vi "Read Configuration Parameters.vi"(8 "error in (no error)":errorcluster, 10 "refnum":T1, 11 "UserPwd DB Configuration in":refnum<class "UserPwd DB Configuration.lvclass">) -> (0 "error out":errorcluster, 2 "refnum out":T1, 3 "UserPwd DB Configuration out":refnum<class "UserPwd DB Configuration.lvclass">)   [LabVIEW 2016, in "UserPwd DB.lvlib" / "UserPwd DB Configuration.lvclass"]
uses:
  <userlib>/Common Components/UserPwd DB/UserPwd DB Config/UserPwd DB Configuration.lvclass
  <vilib>/Utility/config.llb/Config Data RefNum.ctl
  <userlib>/Common Components/UserPwd DB/UserPwd DB/UserPwd DB.lvclass
  <userlib>/Common Components/UserPwd DB/UserPwd DB Config/UserPwd DB Configuration.lvclass/UserPwd DB Configuration.ctl
  <userlib>/Configuration Dialog Actor/Configuration.lvclass
  <vilib>/Utility/config.llb/NI_LVConfig.lvlib
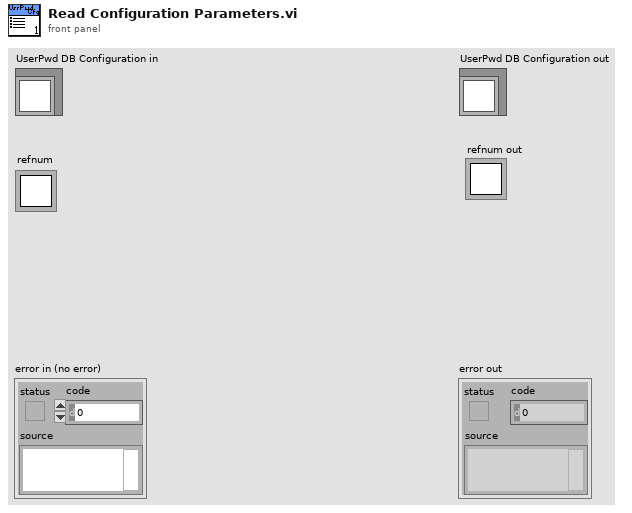
[diagram p1: front panel]
types:
  T1 = typedef "NI_LVConfig.lvlib/Config Data RefNum.ctl" = refnum<k1>
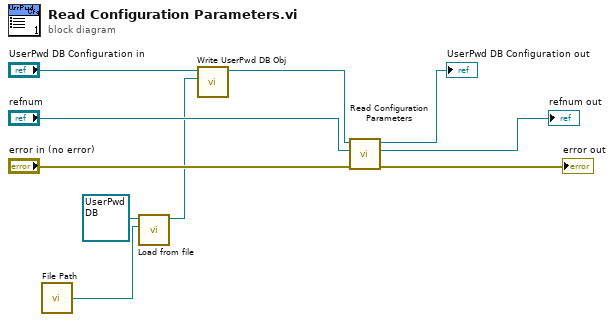
[diagram p0: block diagram]
diagram:
  n1 = call <userlib>:"File Path.vi"() -> ("file path"=w1:path)
  n2 = call <userlib>:"Load from file.vi"("file path (use dialog)"=w1, "UserPwd DB in"=refnum<class "UserPwd DB.lvclass"> refnum) -> ("UserPwd DB out"=w3:refnum<class "UserPwd DB.lvclass">)  [unwired: 8 in, 1 out]
  n3 = call <userlib>:"Write UserPwd DB Obj.vi"("UserPwd DB.lvlib:UserPwd DB.lvclass"=w3, "UserPwd DB Configuration in"="UserPwd DB Configuration in") -> ("UserPwd DB Configuration out"=w4:refnum<class "UserPwd DB Configuration.lvclass">)  [unwired: 9 in]
  n4 = call-parent "Read Configuration Parameters.vi"("error in (no error)"="error in (no error)", "refnum"="refnum", "Configuration in"=w4) -> ("error out"=→"error out":errorcluster, "refnum out"=→"refnum out":T1, "Configuration out"=→"UserPwd DB Configuration out":refnum<class "UserPwd DB Configuration.lvclass">)  [unwired: 6 in]
